vi "S2C_FPGA_DoubleToI16.vi"(4 "Double In":dbl min=-10.0 max=10.0 step=0.0003 format="%#.6g") -> (1 "I16 Out":i16 format="%x")   [LabVIEW 2015]
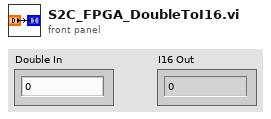
[diagram p1: front panel]
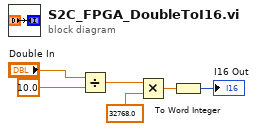
[diagram p0: block diagram]
diagram:
  n1 = Divide(x="Double In", y=sgl 10.0) -> (x/y=w5:dbl)
  n2 = Multiply(x=w5, y=sgl 32768.0) -> (x*y=w3:dbl)
  n3 = To Word Integer(number=w3) -> (16bit integer=→"I16 Out":i16)
